vi "HOST.vi"() -> ()   [LabVIEW 2018]
uses:
  <vilib>/userdefined/High Color/nirio_resource_hc.ctl
  <instrlib>/niDCPower/nidcpower.llb/niDCPower Measurement Type.ctl
  <vilib>/FPGAPlugInAG/PXI-7841R/niLvFpga_Open_PXI-7841R.vi
  <vilib>/rvi/interface/common/dynamic/niFpgaDynamicAddResources.vi
  <vilib>/FPGAPlugInAG/Dynamic/niLvFpga_Reset_Dynamic.vi
  <vilib>/FPGAPlugInAG/Dynamic/niLvFpga_Run_Dynamic.vi
  <vilib>/Utility/error.llb/Error Cluster From Error Code.vi
  <vilib>/rvi/errors/niLvFpgaAdjustHostInterfaceError.vi
  <vilib>/FPGAPlugInAG/Dynamic/niLvFpga_Close_Dynamic.vi
  <vilib>/rvi/interface/nirviOpenFPGA/nirviOpenFPGA.xnode
  FPGA Bitfiles/iCLNGNQI_FPGATarget_Target_OrC3no1FGAk.lvbitx
  <vilib>/rvi/interface/nirviMethod/nirviMethod.xnode
  <vilib>/rvi/interface/nirviReadWriteControl/nirviReadWriteControl.xnode
  <vilib>/rvi/interface/nirviCloseFPGA/nirviCloseFPGA.xnode
  NiFpgaLv.dll
  <vilib>/rvi/interface/Simulation/niFpgaSimulationCallBeginRW.vi
panel:
  in  "Tab Control":T1(tab)
  in  "Проверка ФС NQI":bool
  out "SEL_NQI":bool
  in  "Стоп":bool
  in  "POWER_NQI":bool
  out "SEL_LNG":bool
  in  "SIM_SEL":bool
  in  "Период, мс":u32=1
  out "VDDA_NQI":u32
  out "VDD_NQI":u32
  out "LNG":u32
  out "VDDA_NQI":bool
  out "VDD_NQI":bool
  out "LNG":bool
  in  "VDDA_NQI_selcur":dbl=0.02 caption="current limit" format="%_6p"
  in  "VDD_NQI_selcur":dbl=0.03 caption="current limit" format="%_6p"
  in  "LNG_selcur":dbl=0.06 caption="current limit" format="%_6p"
  in  "POWER_LNG":bool
  in  "VDDA_NQI, V":dbl=4.999999999999997 caption="voltage level" format="%_6p"
  in  "VDDA_NQI_curlim, A":dbl=0.05 caption="current limit" format="%_6p"
  out "VDDA_NQI_cur, A":dbl caption="measurement" format="%_6g"
  out "VDDA_NQI Chart":dbl(graph)=-0.012572351308283002
  in  "VDDA_LNG, V":dbl=5.0 caption="voltage level" format="%_6p"
  in  "VDDA_LNG_curlim, A":dbl=0.1 caption="current limit" format="%_6p"
  in  "VDD_LNG_curlim, A":dbl=0.1 caption="current limit" format="%_6p"
  out "VDDA_LNG_cur, A":dbl caption="measurement" format="%_6g"
  out "VDD_LNG_cur, A":dbl caption="measurement" format="%_6g"
  in  "VDD_LNG, V":dbl=3.3 caption="voltage level" format="%_6p"
  in  "VDD_NQI, V":dbl=4.999999999999997 caption="voltage level" format="%_6p"
  in  "VDD_NQI_curlim, A":dbl=0.1 caption="current limit" format="%_6p"
  out "VDD_NQI_cur, A":dbl caption="measurement" format="%_6g"
  out "VDD_LNG_Chart":dbl(graph)=-0.013606787834847102
  out "VDD_NQI Chart":dbl(graph)=0.03214149952813084
  out "VDDA_LNG_Chart":dbl(graph)=0.06121046446435751 caption="Waveform Chart 5"
  in  "VDDA_VDD_LNG":refnum<k15>="PXI1Slot2" caption="instrument handle"
  in  "VDD_VDDA_NQI":refnum<k15>="PXI1Slot3" caption="instrument handle"
  in  "resource name":T2="PXI1Slot6"
  in  "SEL":path=path "C:/LabView_PRJ/iC_LNG_NQI/SEL"
  out "Номер образца":string="0"
  out "LED_cur, A":dbl caption="measurement" format="%_6g"
  out "LED_Chart":dbl(graph)=0.0008347661178207256
  in  "LED":bool caption="output enabled"
  in  "LED_cl, A":dbl=0.01 caption="current limit" format="%.6p"
  in  "LED, V":dbl=-5.0 caption="voltage level" format="%.6p"
  in  "Мигаем?":bool caption="output enabled"
  out "ERR":i16
  out "NERR":bool
  in  "LED, ms":u32=500
  out "Сумма, мА":dbl
  in  "SEU":path=path "C:/LabView_PRJ/iC_LNG_NQI/SEU"
  in  "Проверка ОС LNG":bool
  out "СБОЙ last":string="ОК"
  out "Сбои":i32
  out "Waveform Chart":cluster{dbl, dbl, dbl, dbl}(graph)={-0.294189453125, -0.3173828125, -0.3009033203125, -0.313720703125}
  out "Сбои NQI":i32
  out "СБОЙ last NQI":string="ОК"
  in  "Сверочный массив":bool[][](array[boolean])=[[FALSE, FALSE, FALSE, FALSE, FALSE, TRUE, FALSE, TRUE], [FALSE, FALSE, FALSE, FALSE, FALSE, TRUE, FALSE, TRUE], [FALSE, FALSE, FALSE, FALSE, FALSE, FALSE, TRUE, TRUE], [FALSE, FALSE, FALSE, FALSE, FALSE, FALSE, TRUE, TRUE], [FALSE, FALSE, FALSE, FALSE, FALSE, FALSE, TRUE, TRUE], [FALSE, FALSE, FALSE, FALSE, FALSE, FALSE, TRUE, TRUE], [FALSE, FALSE, FALSE, FALSE, FALSE, TRUE, FALSE, TRUE], [TRUE, FALSE, FALSE, FALSE, FALSE, FALSE, FALSE, TRUE], [FALSE, TRUE, TRUE, FALSE, TRUE, FALSE, FALSE, TRUE]]
  in  "На чтение":bool[][](array[boolean])=[[FALSE, FALSE, FALSE, FALSE, FALSE, FALSE, FALSE, FALSE, FALSE, FALSE, FALSE, FALSE, FALSE, FALSE, FALSE, FALSE, FALSE, TRUE, FALSE, TRUE, FALSE, FALSE, FALSE, TRUE], [FALSE, FALSE, FALSE, FALSE, FALSE, FALSE, FALSE, FALSE, TRUE, FALSE, FALSE, FALSE, FALSE, FALSE, FALSE, FALSE, FALSE, TRUE, FALSE, TRUE, FALSE, FALSE, FALSE, TRUE], [FALSE, FALSE, FALSE, FALSE, FALSE, FALSE, FALSE, FALSE, FALSE, TRUE, FALSE, FALSE, FALSE, FALSE, FALSE, FALSE, FALSE, TRUE, FALSE, TRUE, FALSE, FALSE, FALSE, TRUE], [FALSE, FALSE, FALSE, FALSE, FALSE, FALSE, FALSE, FALSE, TRUE, TRUE, FALSE, FALSE, FALSE, FALSE, FALSE, FALSE, FALSE, TRUE, FALSE, TRUE, FALSE, FALSE, FALSE, TRUE], [FALSE, FALSE, FALSE, FALSE, FALSE, FALSE, FALSE, FALSE, FALSE, FALSE, TRUE, FALSE, FALSE, FALSE, FALSE, FALSE, FALSE, TRUE, FALSE, TRUE, FALSE, FALSE, FALSE, TRUE], [FALSE, FALSE, FALSE, FALSE, FALSE, FALSE, FALSE, FALSE, TRUE, FALSE, TRUE, FALSE, FALSE, FALSE, FALSE, FALSE, FALSE, TRUE, FALSE, TRUE, FALSE, FALSE, FALSE, TRUE], [FALSE, FALSE, FALSE, FALSE, FALSE, FALSE, FALSE, FALSE, FALSE, TRUE, TRUE, FALSE, FALSE, FALSE, FALSE, FALSE, FALSE, TRUE, FALSE, TRUE, FALSE, FALSE, FALSE, TRUE], [FALSE, FALSE, FALSE, FALSE, FALSE, FALSE, FALSE, FALSE, TRUE, TRUE, TRUE, FALSE, FALSE, FALSE, FALSE, FALSE, FALSE, TRUE, FALSE, TRUE, FALSE, FALSE, FALSE, TRUE], [FALSE, FALSE, FALSE, FALSE, FALSE, FALSE, FALSE, FALSE, FALSE, FALSE, FALSE, TRUE, FALSE, FALSE, FALSE, FALSE, FALSE, TRUE, FALSE, TRUE, FALSE, FALSE, FALSE, TRUE]]
  out "MISO":bool[](array[boolean])
  in  "MOSI":bool[](array[boolean])=[TRUE, TRUE, FALSE, FALSE, FALSE, FALSE, FALSE, TRUE, FALSE, FALSE, FALSE, FALSE, TRUE, TRUE, FALSE, TRUE, FALSE, FALSE, FALSE, FALSE, FALSE, FALSE, FALSE, FALSE]
  in  "N (24/16)":i32=16
  in  "Прошивка":bool
  out "Прошиты!":bool
  out "NSIN":i16
  out "NCOS":i16
  out "PCOS":i16
  out "PSIN":i16
  in  "phase offset N":fxp<+,32,0>
  in  "phase offset P":fxp<+,32,0>
  in  "frequency P":fxp<+,32,0>=2.491287887096405e-08
  in  "frequency N":fxp<+,32,0>=2.491287887096405e-08
  in  "CLKDAT ticks":u16=300
  out "DAT":bool[](array[boolean])
  out "DAT10":bool[](array[boolean])
  out "A":bool
  in  "Offset":i16=10000
  in  "Частота":bool
  in  "NPRG":bool
  in  "CLKDAT":bool
  out "DAT10":u16
  # "Смотрим сумму по ПМ"
  # "LNG"
  # "NQI"
  # "0"
  # "1"
  # "2"
  # "3"
  # "4"
  # "5"
  # "6"
  # "7"
  # "0"
  # "1"
  # "2"
  # "3"
  # "4"
  # "5"
  # "6"
  # "7"
  # "0"
  # "1"
  # "2"
  # "3"
  # "4"
  # "5"
  # "6"
  # "7"
  # "0"
  # "1"
  # "2"
  # "3"
  # "4"
  # "5"
  # "6"
  # "7"
  # "0"
  # "1"
  # "2"
  # "3"
  # "4"
  # "5"
  # "6"
  # "7"
  # "0"
  # "1"
  # "2"
  # "3"
  # "4"
  # "5"
  # "6"
  # "7"
  # "ADDRESS"
  # "DATA"
  # "OPCODE"
  # "0 - программирование"
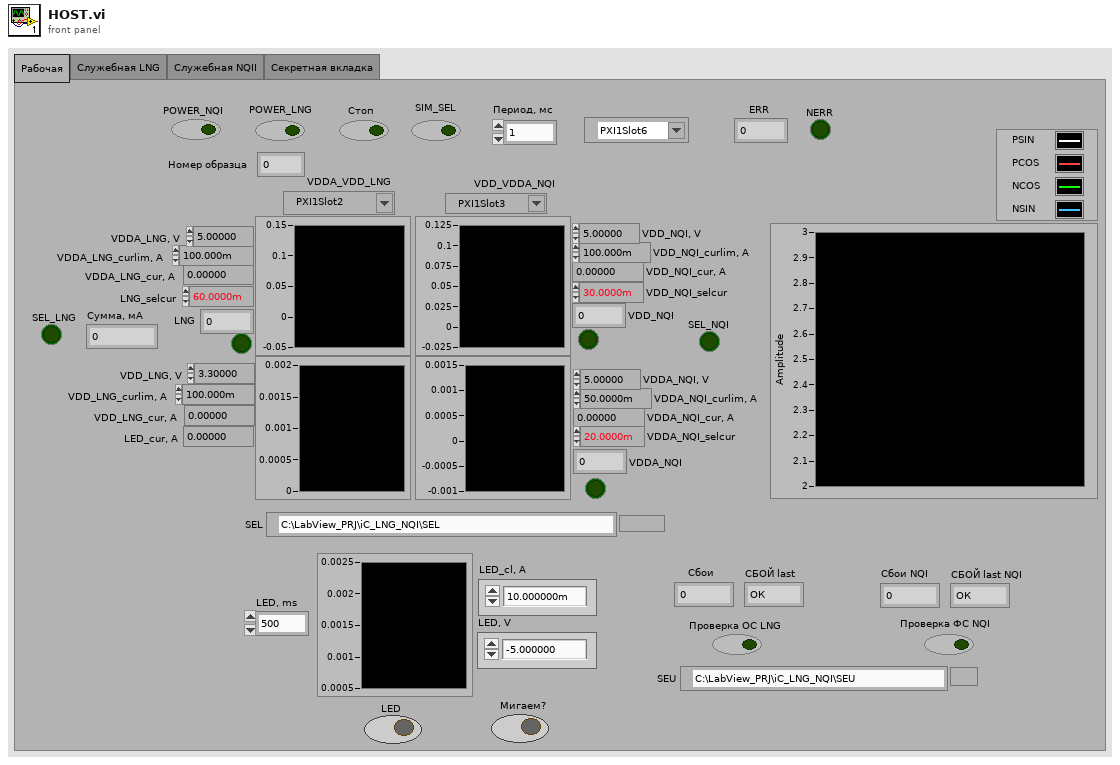
[diagram p1: front panel]
types:
  T1 = enum32{"Рабочая", "Служебная LNG", "Служебная NQII", "Секретная вкладка"}
  T2 = typedef "nirio_resource_hc.ctl" = tag
  T3 = enum16{"open", "replace", "create", "open or create", "replace or create", "replace or create with confirmation"}
  T4 = typedef "niDCPower Measurement Type.ctl" = i32
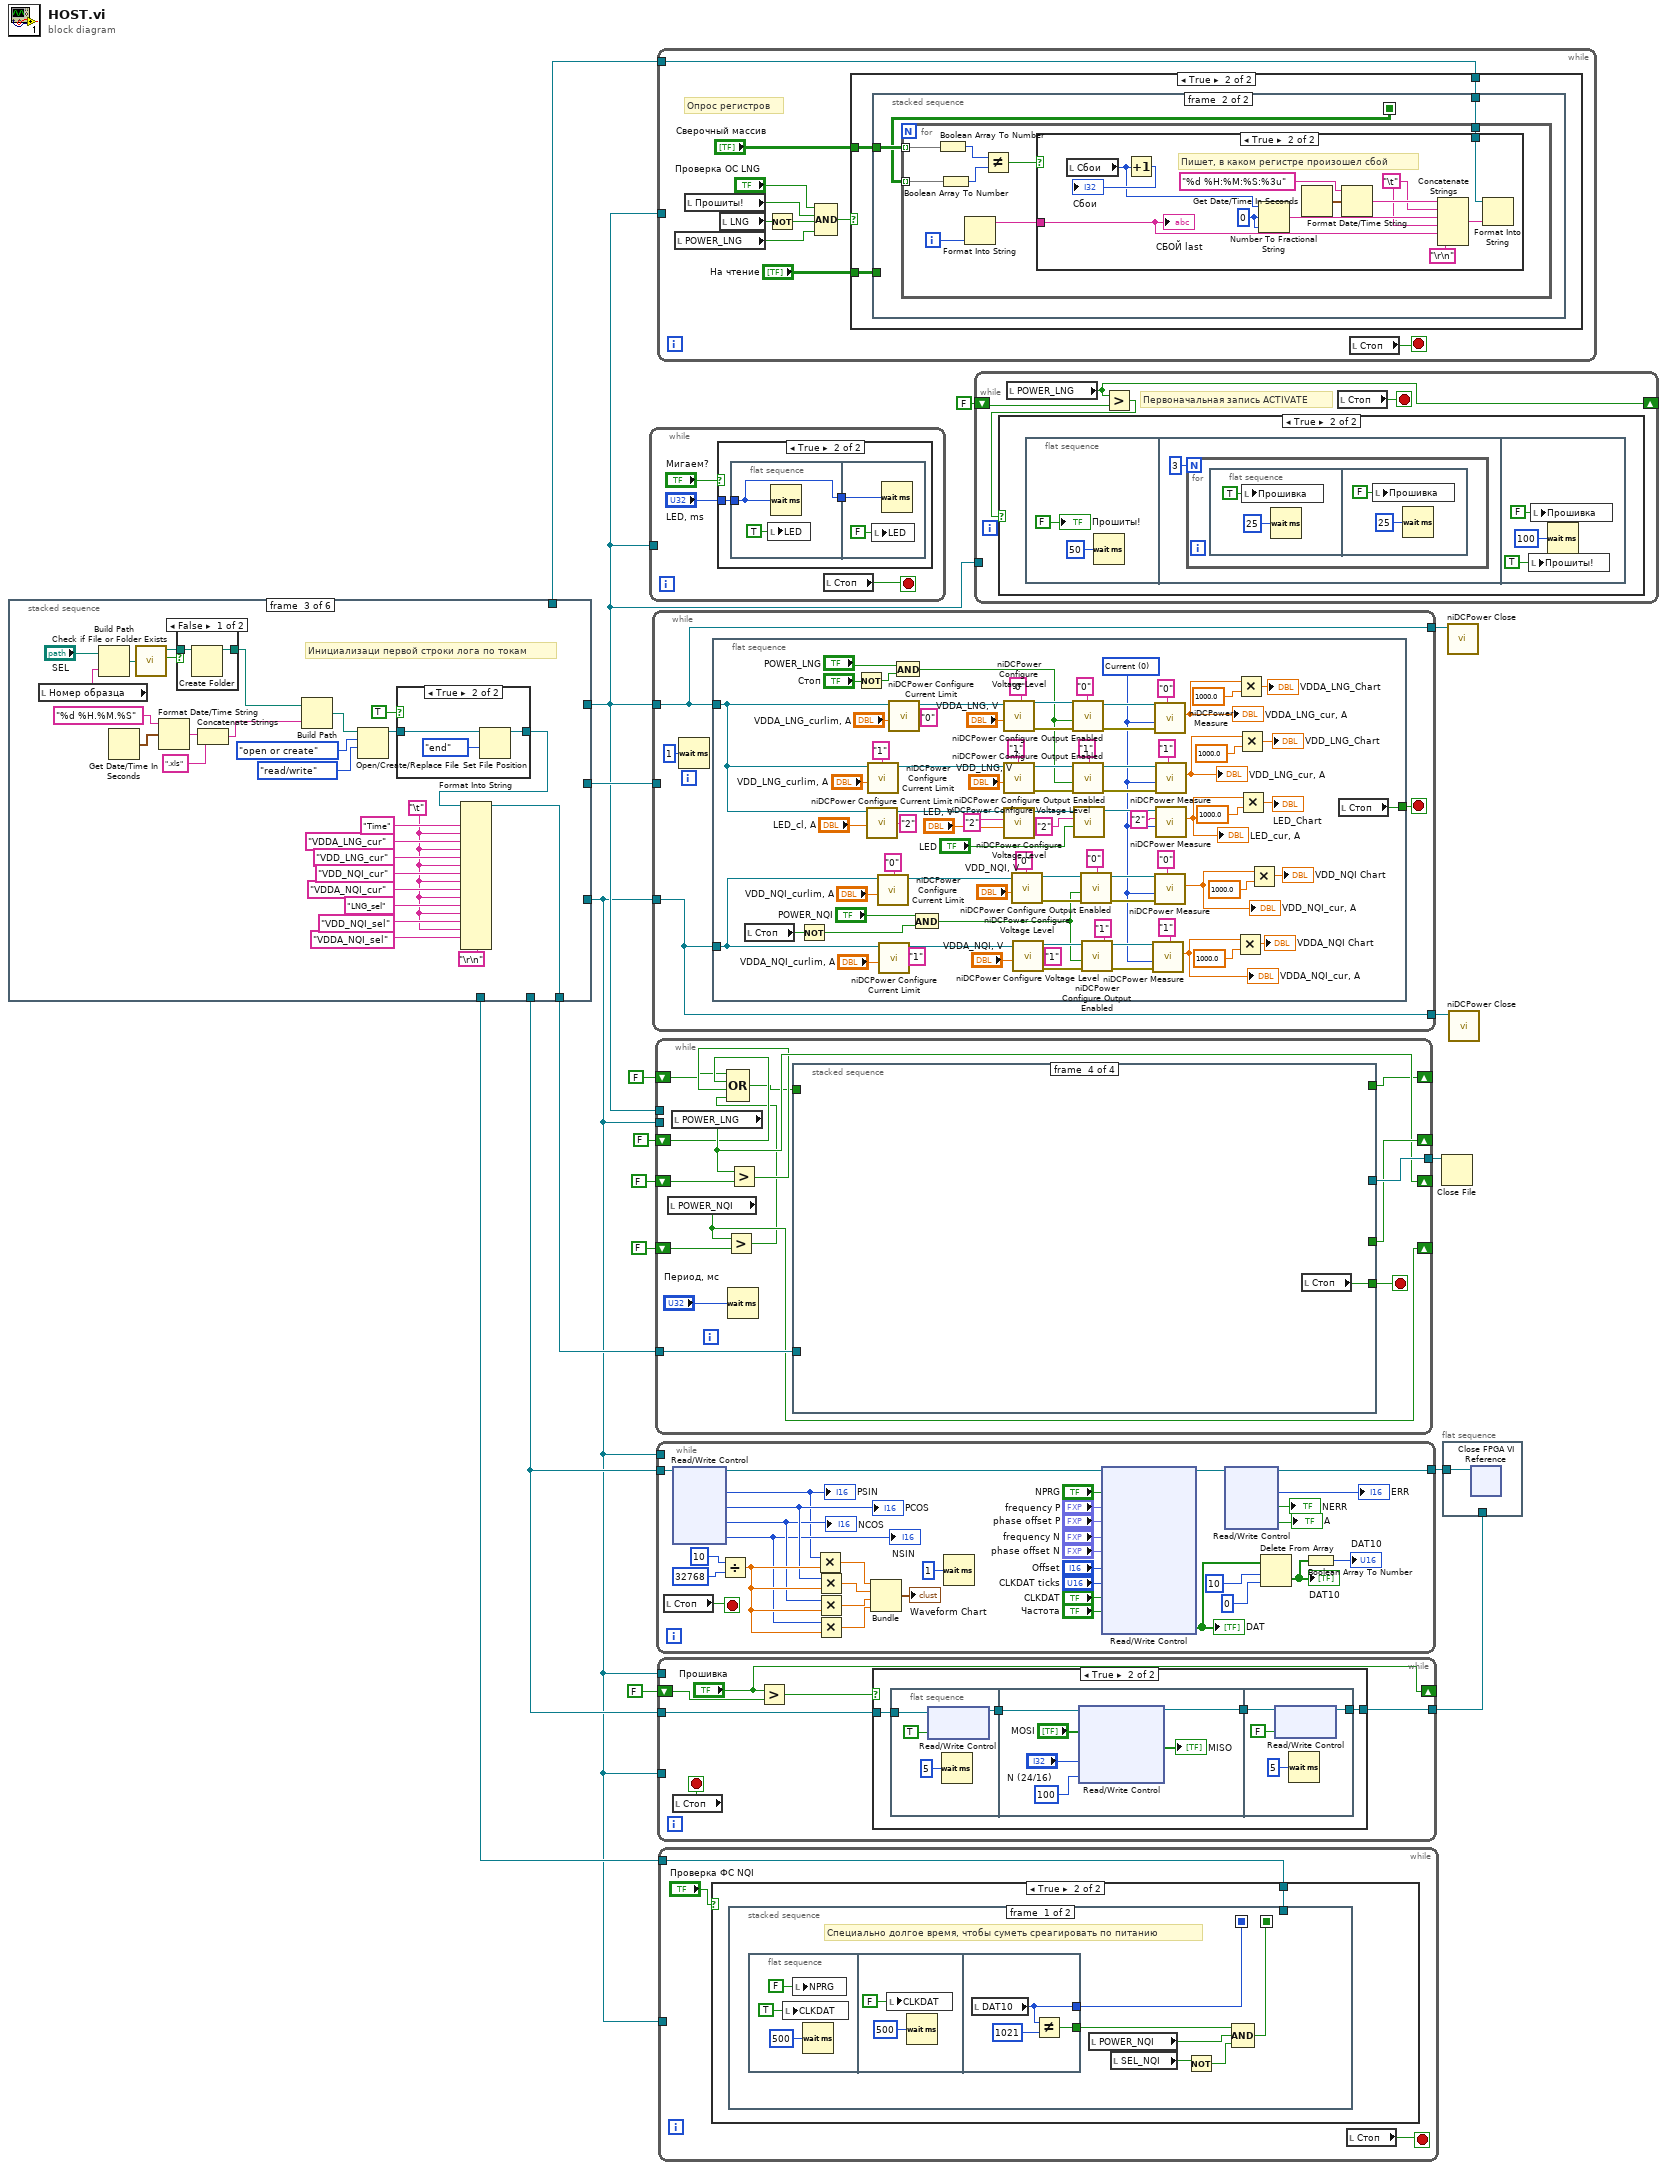
[diagram p0: block diagram]
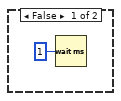
[diagram p2: hidden frame]
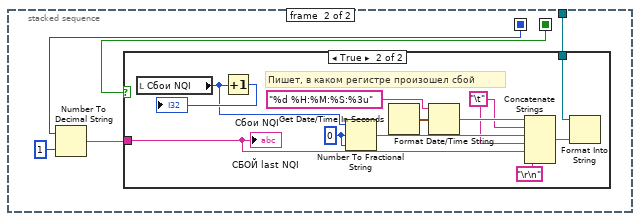
[diagram p3: hidden frame]
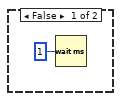
[diagram p5: hidden frame]
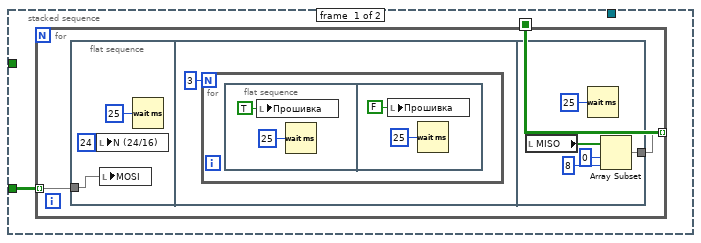
[diagram p6: hidden frame]
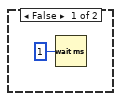
[diagram p8: hidden frame]
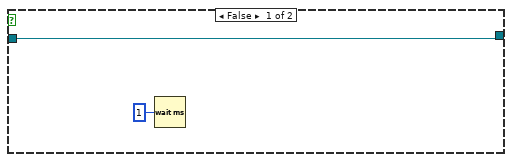
[diagram p9: hidden frame]
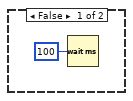
[diagram p10: hidden frame]
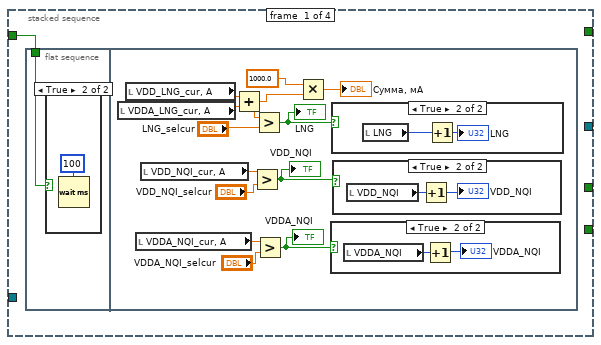
[diagram p11: hidden frame]
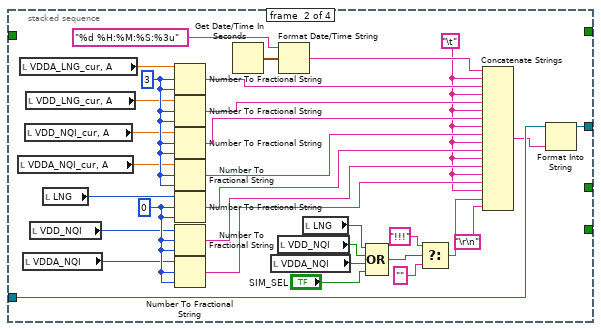
[diagram p16: hidden frame]
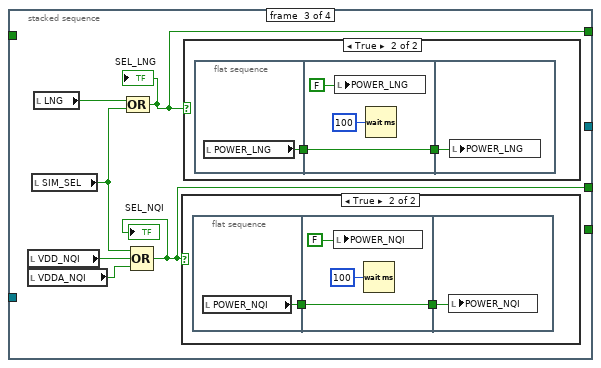
[diagram p17: hidden frame]
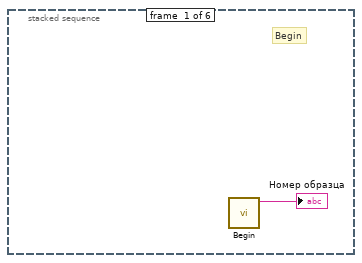
[diagram p20: hidden frame]
diagram:
  n1 = stacked-sequence {
    tunnel: [_ _ w32 _ _ _] -> w15
    tunnel: [_ _ _ _ w93 _] -> w16
    tunnel: [_ _ _ _ _ w100] -> w8
    tunnel: [_ _ _ _ _ w99] -> w5
    tunnel: [_ _ _ _ w93 _] -> w13
    tunnel: [_ _ _ w63 _ _] -> w9
    tunnel: [_ _ _ w63 _ _] -> w6
    frame #0 {
      # "Begin"
      n2 = call "Begin.vi"() -> ("Номер образца 2"=→"Номер образца":string)  [unwired: 11 in]
    }
    frame #1 {
      w21 = "ОК" ("СБОЙ")
      w20 = 0 ("Сбои")
      w27 = u32 0
      w22 = FALSE
      # "Обнуление"
      n3 = local write "LNG"(w22) -> ()
      n4 = local write "VDD_NQI"(w22) -> ()
      n5 = local write "POWER_LNG"(w22) -> ()
      n6 = local write "VDDA_NQI"(w22) -> ()
      n7 = local write "SIM_SEL"(w22) -> ()
      n8 = local write "SEL_LNG"(w22) -> ()
      n9 = local write "POWER_NQI"(w22) -> ()
      n10 = local write "Мигаем?"(w22) -> ()
      n11 = local write "Стоп"(w22) -> ()
      n12 = local write "LED"(w22) -> ()
      n13 = local write "NPRG"(w22) -> ()
      n14 = local write "Частота"(w22) -> ()
      n15 = local write "CLKDAT"(w22) -> ()
      n16 = local write "Проверка ФС NQI"(w22) -> ()
      n17 = local write "N (24/16)"(16 ("N (24/16)")) -> ()
      n18 = local write "MOSI"(bool[] [TRUE, TRUE, FALSE, FALSE, FALSE, FALSE, FALSE, TRUE, FALSE, FALSE, FALSE, FALSE, TRUE, TRUE, FALSE, TRUE, FALSE, FALSE, FALSE, FALSE, FALSE, FALSE, FALSE, FALSE] ("MOSI")) -> ()
      n19 = local write "Проверка ОС LNG"(FALSE ("Проверка сбоев")) -> ()
      n20 = local write "Прошиты!"(FALSE ("Прошиты!")) -> ()
      n21 = local write "LNG"(w27) -> ()
      n22 = local write "VDD_NQI"(w27) -> ()
      n23 = local write "VDDA_NQI"(w27) -> ()
      n24 = local write "Сбои"(w20) -> ()
      n25 = local write "СБОЙ last"(w21) -> ()
      n26 = local write "СБОЙ last NQI"(w21) -> ()
      n27 = local write "Сбои NQI"(w20) -> ()
    }
    frame #2 {
      w30 = "\t"
      # "Инициализаци первой строки лога по токам"
      n28 = local read "Номер образца"() -> (w37:string)
      n29 = Build Path(base path="SEL", name or relative path=w37) -> (appended path=w35:path)
      n30 = Get Date/Time In Seconds() -> (seconds since 1Jan1904=w42:timestamp)
      n31 = call <vilib>:"Check if File or Folder Exists.vi"("path"=w35) -> ("file or folder exists?"=w34:bool, "dup path"=w33:path)  [unwired: 8 in, 1 out]
      n32 = Format Date/Time String(time format string (%c)="%d %H.%M.%S", seconds (now)=w42) -> (date/time string=w45:string)  [unwired: 1 in]
      n33 = case shown="False" w34 {
        tunnel: w33 -> [w61 w62]
        tunnel: [w60 w62] -> w49
        frame False {
          n34 = Create Folder(path (use dialog)=w61) -> (created path=w60:path)  [unwired: 2 in, 2 out]
        }
        frame True {
        }
      }
      n35 = Concatenate Strings(w45, ".xls" ("string")) -> (w47:string)
      n36 = Build Path(base path=w49, name or relative path=w47) -> (appended path=w44:path)
      n37 = Open/Create/Replace File(file path (use dialog)=w44, operation (0:open)=T3."open or create", access (0:read/write)=enum16{"read/write", "read-only", "write-only"}."read/write") -> (refnum out=w41:refnum<file>)  [unwired: 3 in, 2 out]
      n38 = case shown="True" TRUE {
        tunnel: w41 -> [w56 w59]
        tunnel: [w56 w57] -> w48
        frame False {
        }
        frame True {
          n39 = Set File Position(refnum=w59, from (0:start)=enum16{"start", "end", "current"}."end") -> (refnum out=w57:refnum<file>)  [unwired: 2 in, 1 out]
        }
      }
      n40 = Format Into String(initial string=w48, "Time" ("input 1"), w30, "VDDA_LNG_cur" ("input 1"), w30, "VDD_LNG_cur" ("input 1"), w30, "VDD_NQI_cur" ("input 1"), w30, "VDDA_NQI_cur" ("input 1"), w30, "LNG_sel" ("input 1"), w30, "VDD_NQI_sel" ("input 1"), w30, "VDDA_NQI_sel" ("input 1"), "\r\n") -> (resulting string=w32:refnum<file>)  [unwired: 2 in, 1 out]
    }
    frame #3 {
      w76 = "\t"
      # "Логи SEU"
      n41 = local read "Номер образца"() -> (w68:string)
      n42 = Build Path(base path="SEU", name or relative path=w68) -> (appended path=w66:path)
      n43 = Get Date/Time In Seconds() -> (seconds since 1Jan1904=w70:timestamp)
      n44 = call <vilib>:"Check if File or Folder Exists.vi"("path"=w66) -> ("file or folder exists?"=w65:bool, "dup path"=w64:path)  [unwired: 8 in, 1 out]
      n45 = Format Date/Time String(time format string (%c)="%d %H.%M.%S", seconds (now)=w70) -> (date/time string=w72:string)  [unwired: 1 in]
      n46 = case shown="False" w65 {
        tunnel: w64 -> [w91 w92]
        tunnel: [w90 w92] -> w85
        frame False {
          n47 = Create Folder(path (use dialog)=w91) -> (created path=w90:path)  [unwired: 2 in, 2 out]
        }
        frame True {
        }
      }
      n48 = Concatenate Strings(w72, ".xls" ("string")) -> (w73:string)
      n49 = Build Path(base path=w85, name or relative path=w73) -> (appended path=w71:path)
      n50 = Open/Create/Replace File(file path (use dialog)=w71, operation (0:open)=T3."open or create", access (0:read/write)=enum16{"read/write", "read-only", "write-only"}."read/write") -> (refnum out=w69:refnum<file>)  [unwired: 3 in, 2 out]
      n51 = case shown="True" TRUE {
        tunnel: w69 -> [w86 w89]
        tunnel: [w86 w87] -> w74
        frame False {
        }
        frame True {
          n52 = Set File Position(refnum=w89, from (0:start)=enum16{"start", "end", "current"}."end") -> (refnum out=w87:refnum<file>)  [unwired: 2 in, 1 out]
        }
      }
      n53 = Format Into String(initial string=w74, "Time" ("input 1"), w76, "Count" ("input 3"), w76, "#reg" ("input 5"), "\r\n") -> (resulting string=w63:refnum<file>)  [unwired: 2 in, 1 out]
    }
    frame #4 {
      n54 = xnode "Open FPGA VI Reference"("resource name"="resource name") -> ("FPGA VI Reference Out"=w94:refnum<k20>, "error out"=w96:errorcluster)  [unwired: 1 in]
      n55 = xnode "Invoke Method"("FPGA VI Reference In"=w94, "error in"=w96) -> ("FPGA VI Reference Out"=w97:refnum<k20>, "error out"=w95:errorcluster)
      n56 = xnode "Invoke Method"("FPGA VI Reference In"=w97, "error in"=w95) -> ("FPGA VI Reference Out"=w93:refnum<k20>)  [unwired: 1 in, 1 out]
    }
    frame #5 {
      n57 = call <instrlib>:"niDCPower Initialize.vi"("resource name"="VDDA_VDD_LNG") -> ("error out"=w104:errorcluster, "instrument handle out"=w102:refnum<k15>)  [unwired: 3 in, 6 out]
      n58 = call <instrlib>:"niDCPower Initialize.vi"("resource name"="VDD_VDDA_NQI") -> ("error out"=w103:errorcluster, "instrument handle out"=w101:refnum<k15>)  [unwired: 3 in, 6 out]
      n59 = call <instrlib>:"niDCPower Configure Voltage Level.vi"("error in (no error)"=w104, "voltage level"=0.0, "channel name"="0,1", "instrument handle"=w102) -> ("instrument handle out"=w100:refnum<k15>)  [unwired: 6 in, 1 out]
      n60 = call <instrlib>:"niDCPower Configure Voltage Level.vi"("error in (no error)"=w103, "voltage level"=0.0, "channel name"="0,1", "instrument handle"=w101) -> ("instrument handle out"=w99:refnum<k15>)  [unwired: 6 in, 1 out]
    }
  }
  n61 = while {
    tunnel: w8 -> [_]
    stop <- w112 stop-if-true
    n62 = case shown="True" "Мигаем?" {
      tunnel: "LED, ms" -> [_ w116]
      frame False {
        n63 = Wait (ms)(milliseconds to wait=u32 100) -> ()  [unwired: 1 out]
      }
      frame True {
        n64 = flat-sequence {
          tunnel: w116 -> [w117]
          tunnel: [w117] -> w115
          tunnel: w115 -> [w119]
          frame #0 {
            n65 = local write "LED"(TRUE ("LED")) -> ()
            n66 = Wait (ms)(milliseconds to wait=w117) -> ()  [unwired: 1 out]
          }
          frame #1 {
            n67 = local write "LED"(FALSE ("LED")) -> ()
            n68 = Wait (ms)(milliseconds to wait=w119) -> ()  [unwired: 1 out]
          }
        }
      }
    }
    n69 = local read "Стоп"() -> (w112:bool)
  }
  n70 = while {
    tunnel: w5 -> [w121]
    tunnel: w8 -> [w122]
    tunnel: [w122] -> w17
    tunnel: [w121] -> w18
    tunnel: w16 -> [_]
    stop <- w123 stop-if-true
    n71 = Wait (ms)(milliseconds to wait=u32 1) -> ()  [unwired: 1 out]
    n72 = flat-sequence {
      tunnel: w122 -> [w148]
      tunnel: w121 -> [w152]
      tunnel: [w133] -> w123
      frame #0 {
        w140 = T4 0 items=["Current", "Voltage"] ("measurement type")
        n73 = local read "Стоп"() -> (w131:bool)
        n74 = Not(x=w131) -> (.not. x?=w129:bool)
        n75 = Not(x="Стоп") -> (.not. x?=w126:bool)
        n76 = call <instrlib>:"niDCPower Configure Current Limit.vi"("current limit"="LED_cl, A", "channel name"="2", "instrument handle"=w148) -> ("instrument handle out"=w146:refnum<k15>)  [unwired: 7 in, 1 out]
        n77 = call <instrlib>:"niDCPower Configure Current Limit.vi"("current limit"="VDD_LNG_curlim, A", "channel name"="1", "instrument handle"=w148) -> ("instrument handle out"=w196:refnum<k15>)  [unwired: 7 in, 1 out]
        n78 = call <instrlib>:"niDCPower Configure Current Limit.vi"("current limit"="VDD_NQI_curlim, A", "channel name"="0", "instrument handle"=w152) -> ("instrument handle out"=w178:refnum<k15>)  [unwired: 7 in, 1 out]
        n79 = call <instrlib>:"niDCPower Configure Current Limit.vi"("current limit"="VDDA_NQI_curlim, A", "channel name"="1", "instrument handle"=w152) -> ("instrument handle out"=w157:refnum<k15>)  [unwired: 7 in, 1 out]
        n80 = call <instrlib>:"niDCPower Configure Current Limit.vi"("current limit"="VDDA_LNG_curlim, A", "channel name"="0", "instrument handle"=w148) -> ("instrument handle out"=w195:refnum<k15>)  [unwired: 7 in, 1 out]
        n81 = And(x="POWER_LNG", y=w126) -> (x .and. y?=w125:bool)
        n82 = And(x="POWER_NQI", y=w129) -> (x .and. y?=w128:bool)
        n83 = call <instrlib>:"niDCPower Configure Voltage Level.vi"("voltage level"="VDDA_LNG, V", "channel name"="0", "instrument handle"=w195) -> ("error out"=w188:errorcluster, "instrument handle out"=w191:refnum<k15>)  [unwired: 7 in]
        n84 = call <instrlib>:"niDCPower Configure Voltage Level.vi"("voltage level"="VDD_LNG, V", "channel name"="1", "instrument handle"=w196) -> ("error out"=w189:errorcluster, "instrument handle out"=w190:refnum<k15>)  [unwired: 7 in]
        n85 = call <instrlib>:"niDCPower Configure Voltage Level.vi"("voltage level"="LED, V", "channel name"="2", "instrument handle"=w146) -> ("instrument handle out"=w145:refnum<k15>)  [unwired: 7 in, 1 out]
        n86 = call <instrlib>:"niDCPower Configure Voltage Level.vi"("voltage level"="VDD_NQI, V", "channel name"="0", "instrument handle"=w178) -> ("error out"=w182:errorcluster, "instrument handle out"=w183:refnum<k15>)  [unwired: 7 in]
        n87 = call <instrlib>:"niDCPower Configure Voltage Level.vi"("voltage level"="VDDA_NQI, V", "channel name"="1", "instrument handle"=w157) -> ("error out"=w155:errorcluster, "instrument handle out"=w154:refnum<k15>)  [unwired: 7 in]
        n88 = call <instrlib>:"niDCPower Configure Output Enabled.vi"("error in (no error)"=w188, "output enabled"=w125, "channel name"="0", "instrument handle"=w191) -> ("error out"=w200:errorcluster, "instrument handle out"=w199:refnum<k15>)  [unwired: 6 in]
        n89 = call <instrlib>:"niDCPower Configure Output Enabled.vi"("error in (no error)"=w189, "output enabled"=w125, "channel name"="1", "instrument handle"=w190) -> ("error out"=w201:errorcluster, "instrument handle out"=w202:refnum<k15>)  [unwired: 6 in]
        n90 = call <instrlib>:"niDCPower Configure Output Enabled.vi"("output enabled"="LED", "channel name"="2", "instrument handle"=w145) -> ("instrument handle out"=w144:refnum<k15>)  [unwired: 7 in, 1 out]
        n91 = call <instrlib>:"niDCPower Configure Output Enabled.vi"("error in (no error)"=w182, "output enabled"=w128, "channel name"="0", "instrument handle"=w183) -> ("error out"=w174:errorcluster, "instrument handle out"=w175:refnum<k15>)  [unwired: 6 in]
        n92 = call <instrlib>:"niDCPower Configure Output Enabled.vi"("error in (no error)"=w155, "output enabled"=w128, "channel name"="1", "instrument handle"=w154) -> ("error out"=w160:errorcluster, "instrument handle out"=w159:refnum<k15>)  [unwired: 6 in]
        n93 = call <instrlib>:"niDCPower Measure.vi"("error in (no error)"=w160, "measurement type"=w140, "channel name"="1", "instrument handle"=w159) -> ("measurement"=w163:dbl)  [unwired: 5 in, 2 out]
        "VDDA_NQI_cur, A" <- w163
        n94 = call <instrlib>:"niDCPower Measure.vi"("error in (no error)"=w200, "measurement type"=w140, "channel name"="0", "instrument handle"=w199) -> ("measurement"=w167:dbl)  [unwired: 5 in, 2 out]
        "VDDA_LNG_cur, A" <- w167
        n95 = call <instrlib>:"niDCPower Measure.vi"("error in (no error)"=w174, "measurement type"=w140, "channel name"="0", "instrument handle"=w175) -> ("measurement"=w168:dbl)  [unwired: 5 in, 2 out]
        "VDD_NQI_cur, A" <- w168
        n96 = call <instrlib>:"niDCPower Measure.vi"("error in (no error)"=w201, "measurement type"=w140, "channel name"="1", "instrument handle"=w202) -> ("measurement"=w170:dbl)  [unwired: 5 in, 2 out]
        "VDD_LNG_cur, A" <- w170
        n97 = call <instrlib>:"niDCPower Measure.vi"("measurement type"=w140, "channel name"="2", "instrument handle"=w144) -> ("measurement"=w142:dbl)  [unwired: 6 in, 2 out]
        "LED_cur, A" <- w142
        n98 = Multiply(x=w163, y=1000.0) -> (x*y=→"VDDA_NQI Chart":dbl)
        n99 = Multiply(x=w167, y=1000.0) -> (x*y=→"VDDA_LNG_Chart":dbl)
        n100 = Multiply(x=w170, y=1000.0) -> (x*y=→"VDD_LNG_Chart":dbl)
        n101 = Multiply(x=w142, y=1000.0) -> (x*y=→"LED_Chart":dbl)
        n102 = Multiply(x=w168, y=1000.0) -> (x*y=→"VDD_NQI Chart":dbl)
        n103 = local read "Стоп"() -> (w133:bool)
      }
    }
  }
  n104 = while {
    tunnel: w5 -> [_]
    tunnel: w8 -> [_]
    tunnel: w15 -> [w219]
    tunnel: [w217] -> w7
    shift-right: [w216] -> _
    shift-left: FALSE -> [w211]
    shift-right: [w213] -> _
    shift-left: FALSE ("POWER_NQI") -> [w215]
    shift-right: [w212] -> _
    shift-left: FALSE ("POWER_LNG") -> [w214]
    shift-right: [w207] -> _
    shift-left: FALSE -> [w206]
    stop <- w218 stop-if-true
    n105 = local read "POWER_NQI"() -> (w213:bool)
    n106 = local read "POWER_LNG"() -> (w212:bool)
    n107 = Greater?(x=w213, y=w215) -> (0:w209:bool)
    n108 = Wait (ms)(milliseconds to wait="Период, мс") -> ()  [unwired: 1 out]
    n109 = Greater?(x=w212, y=w214) -> (0:w210:bool)
    n110 = Compound Arithmetic op=OR(w206, w211, w210, w209) -> (w208:bool)
    n111 = stacked-sequence {
      tunnel: w208 -> [w221 _ _ _]
      tunnel: w219 -> [_ w271 _ _]
      tunnel: [_ _ _ w295] -> w218
      tunnel: [_ w243 _ _] -> w217
      tunnel: [_ _ w276 _] -> w216
      tunnel: [_ _ w275 _] -> w207
      frame #0 {
        n112 = flat-sequence {
          tunnel: w221 -> [w222]
          frame #0 {
            n113 = case shown="True" w222 {
              frame False {
              }
              frame True {
                n114 = Wait (ms)(milliseconds to wait=u32 100) -> ()  [unwired: 1 out]
              }
            }
          }
          frame #1 {
            n115 = local read "VDDA_LNG_cur, A"() -> (w228:dbl)
            n116 = local read "VDD_LNG_cur, A"() -> (w229:dbl)
            n117 = local read "VDDA_NQI_cur, A"() -> (w234:dbl)
            n118 = local read "VDD_NQI_cur, A"() -> (w236:dbl)
            n119 = Add(x=w229, y=w228) -> (x+y=w226:dbl)
            n120 = Greater?(x=w236, y="VDD_NQI_selcur") -> (0:w231:bool)
            "VDD_NQI" <- w231
            n121 = Greater?(x=w226, y="LNG_selcur") -> (0:w230:bool)
            "LNG" <- w230
            n122 = Greater?(x=w234, y="VDDA_NQI_selcur") -> (0:w232:bool)
            "VDDA_NQI" <- w232
            n123 = Multiply(x=1000.0 ("y"), y=w226) -> (x*y=→"Сумма, мА":dbl)
            n124 = case shown="True" w232 {
              frame False {
              }
              frame True {
                n125 = local read "VDDA_NQI"() -> (w238:u32)
                n126 = Increment(x=w238) -> (x+1=→"VDDA_NQI":u32)
              }
            }
            n127 = case shown="True" w230 {
              frame False {
              }
              frame True {
                n128 = local read "LNG"() -> (w242:u32)
                n129 = Increment(x=w242) -> (x+1=→"LNG":u32)
              }
            }
            n130 = case shown="True" w231 {
              frame False {
              }
              frame True {
                n131 = local read "VDD_NQI"() -> (w240:u32)
                n132 = Increment(x=w240) -> (x+1=→"VDD_NQI":u32)
              }
            }
          }
        }
      }
      frame #1 {
        w273 = i16 0 ("width (-)")
        w272 = i16 3 ("width (-)")
        w244 = "\t"
        n133 = local read "VDDA_NQI_cur, A"() -> (w266:dbl)
        n134 = local read "VDDA_LNG_cur, A"() -> (w269:dbl)
        n135 = local read "VDDA_NQI"() -> (w246:u32)
        n136 = local read "VDD_NQI_cur, A"() -> (w267:dbl)
        n137 = local read "VDD_LNG_cur, A"() -> (w268:dbl)
        n138 = local read "VDD_NQI"() -> (w247:u32)
        n139 = local read "LNG"() -> (w248:u32)
        n140 = Number To Fractional String(number=w269, width (-)=w272, precision (6)=w272) -> (F-format string=w258:string)  [unwired: 1 in]
        n141 = Number To Fractional String(number=w268, width (-)=w272, precision (6)=w272) -> (F-format string=w257:string)  [unwired: 1 in]
        n142 = Number To Fractional String(number=w267, width (-)=w272, precision (6)=w272) -> (F-format string=w256:string)  [unwired: 1 in]
        n143 = Number To Fractional String(number=w266, width (-)=w272, precision (6)=w272) -> (F-format string=w255:string)  [unwired: 1 in]
        n144 = Number To Fractional String(number=w248, width (-)=w273, precision (6)=w273) -> (F-format string=w254:string)  [unwired: 1 in]
        n145 = Number To Fractional String(number=w247, width (-)=w273, precision (6)=w273) -> (F-format string=w253:string)  [unwired: 1 in]
        n146 = Number To Fractional String(number=w246, width (-)=w273, precision (6)=w273) -> (F-format string=w252:string)  [unwired: 1 in]
        n147 = Get Date/Time In Seconds() -> (seconds since 1Jan1904=w270:timestamp)
        n148 = local read "VDDA_NQI"() -> (w264:bool)
        n149 = local read "VDD_NQI"() -> (w265:bool)
        n150 = Format Date/Time String(time format string (%c)="%d %H:%M:%S:%3u", seconds (now)=w270) -> (date/time string=w259:string)  [unwired: 1 in]
        n151 = local read "LNG"() -> (w245:bool)
        n152 = Compound Arithmetic op=OR(w245, w265, w264, "SIM_SEL") -> (w260:bool)
        n153 = Select(t="!!!", s=w260, f="") -> (s? t:f=w251:string)
        n154 = Concatenate Strings(w259, w244, w258, w244, w257, w244, w256, w244, w255, w244, w254, w244, w253, w244, w252, w244, w251, "\r\n") -> (w249:string)
        n155 = Format Into String(initial string=w271, w249) -> (resulting string=w243:refnum<file>)  [unwired: 2 in, 1 out]
      }
      frame #2 {
        n156 = local read "VDD_NQI"() -> (w278:bool)
        n157 = local read "VDDA_NQI"() -> (w277:bool)
        n158 = local read "SIM_SEL"() -> (w279:bool)
        n159 = local read "LNG"() -> (w280:bool)
        n160 = Compound Arithmetic op=OR(w280, w279) -> (w275:bool)
        "SEL_LNG" <- w275
        n161 = Compound Arithmetic op=OR(w279, w278, w277) -> (w276:bool)
        "SEL_NQI" <- w276
        n162 = case shown="True" w276 {
          frame False {
          }
          frame True {
            n163 = flat-sequence {
              tunnel: [w283] -> w282
              tunnel: [w286] -> w281
              tunnel: w282 -> [w286]
              tunnel: w281 -> [w287]
              frame #0 {
                n164 = local read "POWER_NQI"() -> (w283:bool)
              }
              frame #1 {
                n165 = local write "POWER_NQI"(FALSE) -> ()
                n166 = Wait (ms)(milliseconds to wait=u32 100) -> ()  [unwired: 1 out]
              }
              frame #2 {
                n167 = local write "POWER_NQI"(w287) -> ()
              }
            }
          }
        }
        n168 = case shown="True" w275 {
          frame False {
          }
          frame True {
            n169 = flat-sequence {
              tunnel: [w290] -> w288
              tunnel: [w293] -> w289
              tunnel: w288 -> [w293]
              tunnel: w289 -> [w294]
              frame #0 {
                n170 = local read "POWER_LNG"() -> (w290:bool)
              }
              frame #1 {
                n171 = local write "POWER_LNG"(FALSE) -> ()
                n172 = Wait (ms)(milliseconds to wait=u32 100) -> ()  [unwired: 1 out]
              }
              frame #2 {
                n173 = local write "POWER_LNG"(w294) -> ()
              }
            }
          }
        }
      }
      frame #3 {
        n174 = local read "Стоп"() -> (w295:bool)
      }
    }
  }
  n175 = while {
    tunnel: w5 -> [_]
    tunnel: w13 -> [w328]
    tunnel: [w312] -> w14
    stop <- w329 stop-if-true
    n176 = local read "Стоп"() -> (w329:bool)
    n177 = xnode "Read/Write Control"("FPGA VI Reference In"=w328) -> ("FPGA VI Reference Out"=w315:refnum<k20>, "PSIN"=w316:i16, "PCOS"=w319:i16, "NCOS"=w318:i16, "NSIN"=w317:i16)  [unwired: 1 in, 1 out]
    "PSIN" <- w316
    "PCOS" <- w319
    "NCOS" <- w318
    "NSIN" <- w317
    n178 = Divide(x=10, y=32768) -> (x/y=w325:dbl)
    n179 = Multiply(x=w316, y=w325) -> (x*y=w324:dbl)
    n180 = Multiply(x=w319, y=w325) -> (x*y=w323:dbl)
    n181 = Multiply(x=w318, y=w325) -> (x*y=w322:dbl)
    n182 = Multiply(x=w317, y=w325) -> (x*y=w321:dbl)
    n183 = Bundle(w324, w323, w322, w321) -> (→"Waveform Chart":cluster{dbl, dbl, dbl, dbl})  [unwired: 1 in]
    n184 = Wait (ms)(milliseconds to wait=u32 1) -> ()  [unwired: 1 out]
    n185 = xnode "Read/Write Control"("FPGA VI Reference In"=w315, "NPRG"="NPRG", "frequency P"="frequency P", "phase offset P"="phase offset P", "frequency N"="frequency N", "phase offset N"="phase offset N", "Offset"="Offset", "CLKDAT ticks"="CLKDAT ticks", "CLKDAT"="CLKDAT", "Частота"="Частота") -> ("FPGA VI Reference Out"=w313:refnum<k20>, "DAT"=w298:bool[])  [unwired: 1 in, 1 out]
    "DAT" <- w298
    n186 = xnode "Read/Write Control"("FPGA VI Reference In"=w313) -> ("FPGA VI Reference Out"=w312:refnum<k20>, "ERR"=→"ERR":i16, "NERR"=→"NERR":bool, "A"=→"A":bool)  [unwired: 1 in, 1 out]
    n187 = Delete From Array(array=w298, length=10, index=0) -> (deleted portion=w297:bool[])  [unwired: 1 out]
    "DAT10" <- w297
    n188 = Boolean Array To Number(Boolean array=w297) -> (number=→"DAT10":u16)
  }
  n189 = while {
    tunnel: w9 -> [w331]
    tunnel: w8 -> [_]
    stop <- w340 stop-if-true
    # "Опрос регистров"
    n190 = local read "POWER_LNG"() -> (w335:bool)
    n191 = local read "Прошиты!"() -> (w337:bool)
    n192 = local read "LNG"() -> (w339:bool)
    n193 = Not(x=w339) -> (.not. x?=w336:bool)
    n194 = Compound Arithmetic op=AND("Проверка ОС LNG", w337, w336, w335) -> (w334:bool)
    n195 = case shown="True" w334 {
      tunnel: "Сверочный массив" -> [_ w343]
      tunnel: "На чтение" -> [_ w344]
      tunnel: w331 -> [_ w342]
      frame False {
        n196 = Wait (ms)(milliseconds to wait=u32 1) -> ()  [unwired: 1 out]
      }
      frame True {
        n197 = stacked-sequence {
          seq-local: [w346 _] -> [_ w363]
          tunnel: w344 -> [w345 _]
          tunnel: w343 -> [_ w364]
          tunnel: w342 -> [_ w362]
          frame #0 {
            n198 = for {
              tunnel: [w348] -> w346 mode=indexing
              tunnel: w345 -> [w347] mode=indexing
              n199 = flat-sequence {
                tunnel: w347 -> [w350]
                tunnel: [w358] -> w348
                frame #0 {
                  n200 = local write "N (24/16)"(24 ("N (24/16)")) -> ()
                  n201 = local write "MOSI"(w350) -> ()
                  n202 = Wait (ms)(milliseconds to wait=u32 25) -> ()  [unwired: 1 out]
                }
                frame #1 {
                  n203 = for {
                    N: 3 -> [_]
                    n204 = flat-sequence {
                      frame #0 {
                        n205 = local write "Прошивка"(TRUE ("Прошивка")) -> ()
                        n206 = Wait (ms)(milliseconds to wait=u32 25) -> ()  [unwired: 1 out]
                      }
                      frame #1 {
                        n207 = local write "Прошивка"(FALSE ("Прошивка")) -> ()
                        n208 = Wait (ms)(milliseconds to wait=u32 25) -> ()  [unwired: 1 out]
                      }
                    }
                  }
                }
                frame #2 {
                  n209 = local read "MISO"() -> (w361:bool[])
                  n210 = Wait (ms)(milliseconds to wait=u32 25) -> ()  [unwired: 1 out]
                  n211 = Array Subset(array=w361, index=0, length=8) -> (w358:bool[])
                }
              }
            }
          }
          frame #1 {
            n212 = for {
              tunnel: w364 -> [w372] mode=indexing
              tunnel: w363 -> [w371] mode=indexing
              tunnel: w362 -> [w365]
              i -> [w367]
              n213 = Boolean Array To Number(Boolean array=w372) -> (number=w370:u32)
              n214 = Boolean Array To Number(Boolean array=w371) -> (number=w369:u32)
              n215 = Format Into String(w367) -> (resulting string=w366:string)  [unwired: 3 in, 1 out]
              n216 = Not Equal?(x=w370, y=w369) -> (x != y?=w368:bool)
              n217 = case shown="True" w368 {
                tunnel: w366 -> [_ w376]
                tunnel: w365 -> [_ w373]
                frame False {
                }
                frame True {
                  w380 = i16 0 ("width (-)")
                  w379 = "\t"
                  # "Пишет, в каком регистре произошел сбой"
                  n218 = local read "Сбои"() -> (w374:i32)
                  n219 = Increment(x=w374) -> (x+1=→"Сбои":i32)
                  n220 = Number To Fractional String(number=w374, width (-)=w380, precision (6)=w380) -> (F-format string=w381:string)  [unwired: 1 in]
                  n221 = Get Date/Time In Seconds() -> (seconds since 1Jan1904=w384:timestamp)
                  n222 = Format Date/Time String(time format string (%c)="%d %H:%M:%S:%3u", seconds (now)=w384) -> (date/time string=w383:string)  [unwired: 1 in]
                  n223 = Concatenate Strings(w383, w379, w381, w379, w376, "\r\n") -> (w382:string)
                  n224 = Format Into String(initial string=w373, w382) -> ()  [unwired: 2 in, 2 out]
                  "СБОЙ last" <- w376
                }
              }
            }
          }
        }
      }
    }
    n225 = local read "Стоп"() -> (w340:bool)
  }
  n226 = while {
    tunnel: w13 -> [w389]
    tunnel: w5 -> [_]
    tunnel: [w388] -> w12
    shift-right: ["Прошивка"] -> _
    shift-left: FALSE ("Прошивка") -> [w387]
    tunnel: w5 -> [_]
    stop <- w390 stop-if-true
    n227 = local read "Стоп"() -> (w390:bool)
    n228 = Greater?(x="Прошивка", y=w387) -> (0:w385:bool)
    n229 = case shown="True" w385 {
      tunnel: w389 -> [w391 w396]
      tunnel: [w391 w393] -> w388
      frame False {
        n230 = Wait (ms)(milliseconds to wait=u32 1) -> ()  [unwired: 1 out]
      }
      frame True {
        n231 = flat-sequence {
          tunnel: w396 -> [w400]
          tunnel: [w397] -> w395
          tunnel: w395 -> [w404]
          tunnel: [w403] -> w394
          tunnel: w394 -> [w408]
          tunnel: [w407] -> w393
          frame #0 {
            n232 = xnode "Read/Write Control"("FPGA VI Reference In"=w400, "Регистр"=TRUE) -> ("FPGA VI Reference Out"=w397:refnum<k20>)  [unwired: 1 in, 1 out]
            n233 = Wait (ms)(milliseconds to wait=u32 5) -> ()  [unwired: 1 out]
          }
          frame #1 {
            n234 = xnode "Read/Write Control"("FPGA VI Reference In"=w404, "MOSI"="MOSI", "N (24/16)"="N (24/16)", "Count(Ticks)"=u16 100) -> ("FPGA VI Reference Out"=w403:refnum<k20>, "MISO"=→"MISO":bool[])  [unwired: 1 in, 1 out]
          }
          frame #2 {
            n235 = xnode "Read/Write Control"("FPGA VI Reference In"=w408, "Регистр"=FALSE) -> ("FPGA VI Reference Out"=w407:refnum<k20>)  [unwired: 1 in, 1 out]
            n236 = Wait (ms)(milliseconds to wait=u32 5) -> ()  [unwired: 1 out]
          }
        }
      }
    }
  }
  n237 = while {
    tunnel: w6 -> [w411]
    tunnel: w5 -> [_]
    stop <- w413 stop-if-true
    n238 = case shown="True" "Проверка ФС NQI" {
      tunnel: w411 -> [_ w415]
      frame False {
        n239 = Wait (ms)(milliseconds to wait=u32 1) -> ()  [unwired: 1 out]
      }
      frame True {
        n240 = stacked-sequence {
          seq-local: [w416 _] -> [_ w430]
          seq-local: [w421 _] -> [_ w434]
          tunnel: w415 -> [_ w431]
          frame #0 {
            # "Специально долгое время, чтобы суметь среагировать по питанию"
            n241 = flat-sequence {
              tunnel: [w428] -> w419
              tunnel: [w427] -> w421
              frame #0 {
                n242 = local write "CLKDAT"(TRUE ("CLKDAT")) -> ()
                n243 = local write "NPRG"(FALSE ("NPRG")) -> ()
                n244 = Wait (ms)(milliseconds to wait=u32 500) -> ()  [unwired: 1 out]
              }
              frame #1 {
                n245 = local write "CLKDAT"(FALSE ("CLKDAT")) -> ()
                n246 = Wait (ms)(milliseconds to wait=u32 500) -> ()  [unwired: 1 out]
              }
              frame #2 {
                n247 = local read "DAT10"() -> (w427:u16)
                n248 = Not Equal?(x=w427, y=u16 1021) -> (x != y?=w428:bool)
              }
            }
            n249 = local read "POWER_NQI"() -> (w418:bool)
            n250 = local read "SEL_NQI"() -> (w420:bool)
            n251 = Not(x=w420) -> (.not. x?=w417:bool)
            n252 = Compound Arithmetic op=AND(w419, w418, w417) -> (w416:bool)
          }
          frame #1 {
            n253 = Number To Decimal String(number=w434, width (-)=i16 1) -> (decimal integer string=w432:string)
            n254 = case shown="True" w430 {
              tunnel: w432 -> [_ w438]
              tunnel: w431 -> [_ w435]
              frame False {
              }
              frame True {
                w442 = i16 0 ("width (-)")
                w441 = "\t"
                # "Пишет, в каком регистре произошел сбой"
                n255 = local read "Сбои NQI"() -> (w436:i32)
                n256 = Increment(x=w436) -> (x+1=→"Сбои NQI":i32)
                n257 = Number To Fractional String(number=w436, width (-)=w442, precision (6)=w442) -> (F-format string=w443:string)  [unwired: 1 in]
                n258 = Get Date/Time In Seconds() -> (seconds since 1Jan1904=w446:timestamp)
                n259 = Format Date/Time String(time format string (%c)="%d %H:%M:%S:%3u", seconds (now)=w446) -> (date/time string=w445:string)  [unwired: 1 in]
                n260 = Concatenate Strings(w445, w441, w443, w441, w438, "\r\n") -> (w444:string)
                n261 = Format Into String(initial string=w435, w444) -> ()  [unwired: 2 in, 2 out]
                "СБОЙ last NQI" <- w438
              }
            }
          }
        }
      }
    }
    n262 = local read "Стоп"() -> (w413:bool)
  }
  n263 = while {
    tunnel: w8 -> [_]
    shift-right: [w449] -> _
    shift-left: FALSE ("POWER_LNG") -> [w448]
    stop <- w450 stop-if-true
    # "Первоначальная запись ACTIVATE"
    n264 = local read "POWER_LNG"() -> (w449:bool)
    n265 = Greater?(x=w449, y=w448) -> (0:w447:bool)
    n266 = case shown="True" w447 {
      frame False {
        n267 = Wait (ms)(milliseconds to wait=u32 1) -> ()  [unwired: 1 out]
      }
      frame True {
        n268 = flat-sequence {
          frame #0 {
            n269 = Wait (ms)(milliseconds to wait=u32 50) -> ()  [unwired: 1 out]
            "Прошиты!" <- FALSE ("Прошиты!")
          }
          frame #1 {
            n270 = for {
              N: 3 -> [_]
              n271 = flat-sequence {
                frame #0 {
                  n272 = local write "Прошивка"(TRUE ("Прошивка")) -> ()
                  n273 = Wait (ms)(milliseconds to wait=u32 25) -> ()  [unwired: 1 out]
                }
                frame #1 {
                  n274 = local write "Прошивка"(FALSE ("Прошивка")) -> ()
                  n275 = Wait (ms)(milliseconds to wait=u32 25) -> ()  [unwired: 1 out]
                }
              }
            }
          }
          frame #2 {
            n276 = local write "Прошиты!"(TRUE ("Прошиты!")) -> ()
            n277 = local write "Прошивка"(FALSE ("Прошивка")) -> ()
            n278 = Wait (ms)(milliseconds to wait=u32 100) -> ()  [unwired: 1 out]
          }
        }
      }
    }
    n279 = local read "Стоп"() -> (w450:bool)
  }
  n280 = Close File(refnum=w7) -> ()  [unwired: 1 in, 2 out]
  n281 = flat-sequence {
    tunnel: w14 -> [w462]
    tunnel: w12 -> [_]
    frame #0 {
      n282 = xnode "Close FPGA VI Reference"("FPGA VI Reference In"=w462) -> ()  [unwired: 1 in, 1 out]
    }
  }
  n283 = call <instrlib>:"niDCPower Close.vi"("instrument handle"=w17) -> ()  [unwired: 10 in, 1 out]
  n284 = call <instrlib>:"niDCPower Close.vi"("instrument handle"=w18) -> ()  [unwired: 10 in, 1 out]
